vi "Move API.vi"(8 "Error In":errorcluster, 10 "Wait (ms)":u32) -> (0 "Error Out":errorcluster)   [LabVIEW 2017, in "Shutter.lvlib"]
uses:
  Shutter.lvlib
  Controls/Module Command Data [cluster].ctl
  Controls/Module Commands [enum].ctl
  Events/Events.lvlib
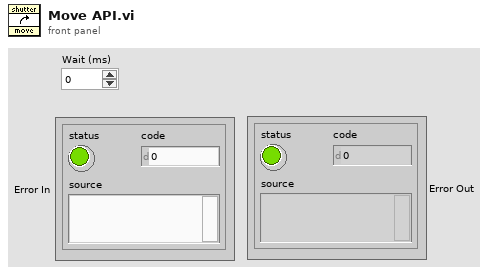
[diagram p1: front panel]
types:
  T1 = typedef "Shutter.lvlib/Module Command Data [cluster].ctl" = cluster{"Command":T2, "Data":variant}
  T2 = typedef "Shutter.lvlib/Module Commands [enum].ctl" = enum16{"Start", "Move", "Return", "Stop"}
  T3 = typedef "Events.lvlib/Refs [cluster].ctl" = cluster{"Exit":refnum<user-event>, "Controller":refnum<user-event>, "System Error":refnum<user-event>, "UI":refnum<user-event>, "Example Module":refnum<user-event>, "Shutter":refnum<user-event>, "Monochromator":refnum<user-event>, "DAQ":refnum<user-event>, "Scope":refnum<user-event>, "Processing":refnum<user-event>, "File IO":refnum<user-event>, "Colour wheel":refnum<user-event>}
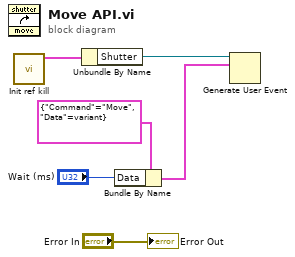
[diagram p0: block diagram]
diagram:
  n1 = call "Init ref kill.vi"() -> ("Messages"=w6:T3)  [unwired: 10 in, 1 out]
  n2 = Unbundle By Name(w6) -> ("Shutter"=w4:refnum<user-event>)
  n3 = Bundle By Name(cluster=T1 {"Command"=enum."Move", "Data"=variant} ("event data"), "Data"="Wait (ms)") -> (w2:T1)
  n4 = Generate User Event(user event=w4, event data cluster=w2) -> ()  [unwired: 2 in, 2 out]
  "Error Out" <- "Error In"
